vi "Write Measurement Name.vi"(8 "error in (no error)":errorcluster, 10 "Measurement Name":string, 11 "SeqAuto IEvaluation in":refnum<class "SeqAuto IEvaluation.lvclass">) -> (0 "error out":errorcluster, 3 "SeqAuto IEvaluation out":refnum<class "SeqAuto IEvaluation.lvclass">)   [LabVIEW 2018, in "IEvaluation.lvlib" / "SeqAuto IEvaluation.lvclass"]
uses:
  SeqAuto IEvaluation.lvclass
  SeqAuto IEvaluation.lvclass/SeqAuto IEvaluation.ctl
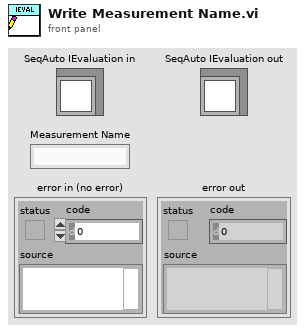
[diagram p1: front panel]
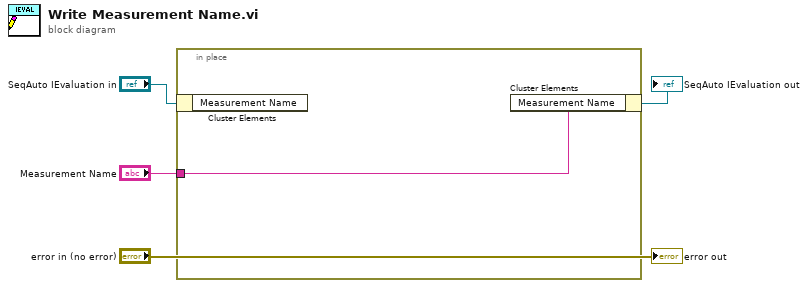
[diagram p0: block diagram]
diagram:
  n1 = in-place {
    in-place-border: "Measurement Name" -> [w5]
    n2 = in-place-cluster #1("SeqAuto IEvaluation in") -> ()  [unwired: 1 out]
    n3 = in-place-cluster #1("Measurement Name"=w5) -> (→"SeqAuto IEvaluation out":refnum<class "SeqAuto IEvaluation.lvclass">)
  }
  "error out" <- "error in (no error)"
